vi "Catapult Controller.vi"(8 "error in (no error)":errorcluster, 9 "De-energize w/out Re-energizing":bool, 10 "Wedge Button":bool, 11 "Catapult Trigger":bool) -> (0 "error out":errorcluster)   [LabVIEW 2013]
uses:
  Systems/Catapult/Catapult.lvclass
  Robot Global Data.vi
  Commands/CT-Energize-Cmd/CT-Energize-Cmd.lvclass
  <vilib>/Rock Robotics/WPI/Solenoid/WPI_SolenoidSetEnum.vi
  <vilib>/Rock Robotics/WPI/Solenoid/WPI_SolenoidValue.ctl
  Commands/CT-Stop-Command/CT-Stop-Cmd.lvclass
  Commands/CT-De-energize-Command/CT-De-energize-Cmd.lvclass
panel:
  in  "Boolean 4":bool
  in  "Boolean 3":bool
  in  "Counter":i8
  # "Disabled (Used in Testing)"
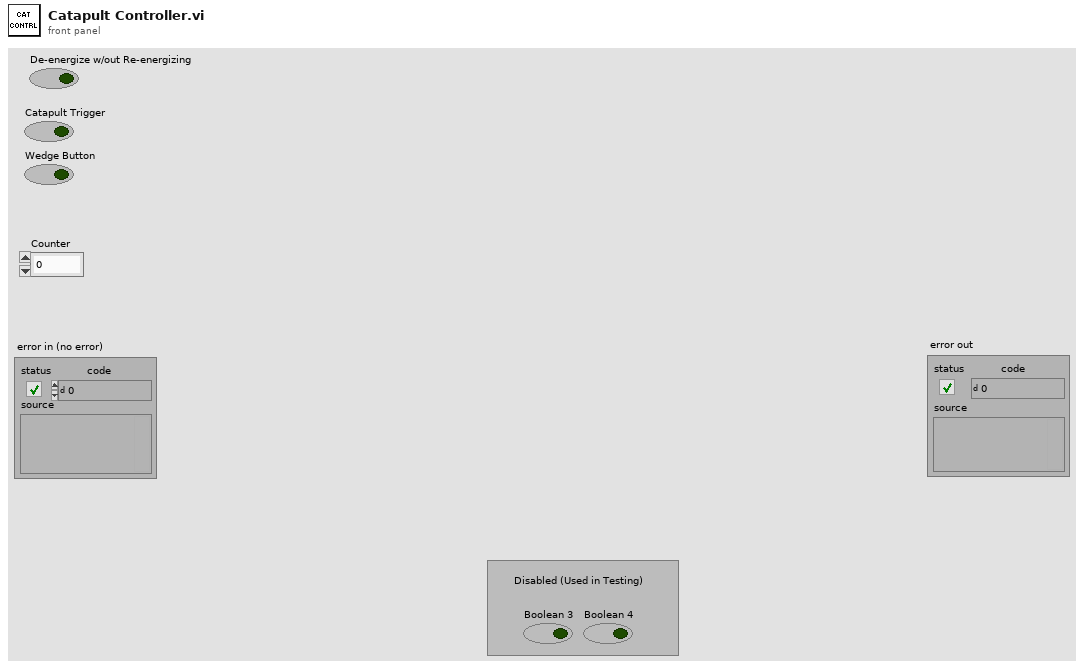
[diagram p1: front panel]
types:
  T1 = typedef "Semaphore RefNum" = refnum<k1>
  T2 = typedef "WPI_DigitalInputDevRef.ctl" = cluster{"DevStatus":errorcluster, "DIO Channel":T3, "Digital Module":T4}
  T3 = typedef "FPGA_DIOChannel.ctl" = enum8{"DIO 1", "DIO 2", "DIO 3", "DIO 4", "DIO 5", "DIO 6", "DIO 7", "DIO 8", "DIO 9", "DIO 10", "DIO 11", "DIO 12", "DIO 13", "DIO 14", "Invalid"}
  T4 = typedef "FPGA_TypedefDigitalModule.ctl" = enum16{"Digital Module 1", "Digital Module 2"}
  T5 = typedef "WPI_SolenoidValue.ctl" = enum16{"Off", "On", "Forward", "Reverse"}
  T6 = typedef "WPI_SolenoidDevRef.ctl" = cluster{"DevStatus":errorcluster, "Solenoid Module":T7, "Forward Solenoid Channel":T8, "Reverse Solenoid Channel":T8}
  T7 = typedef "FPGA_TypedefSolenoidModule.ctl" = enum16{"Solenoid Module 1", "Solenoid Module 2"}
  T8 = typedef "WPI_SolenoidChannel.ctl" = enum8{"Solenoid 1", "Solenoid 2", "Solenoid 3", "Solenoid 4", "Solenoid 5", "Solenoid 6", "Solenoid 7", "Solenoid 8", "Invalid"}
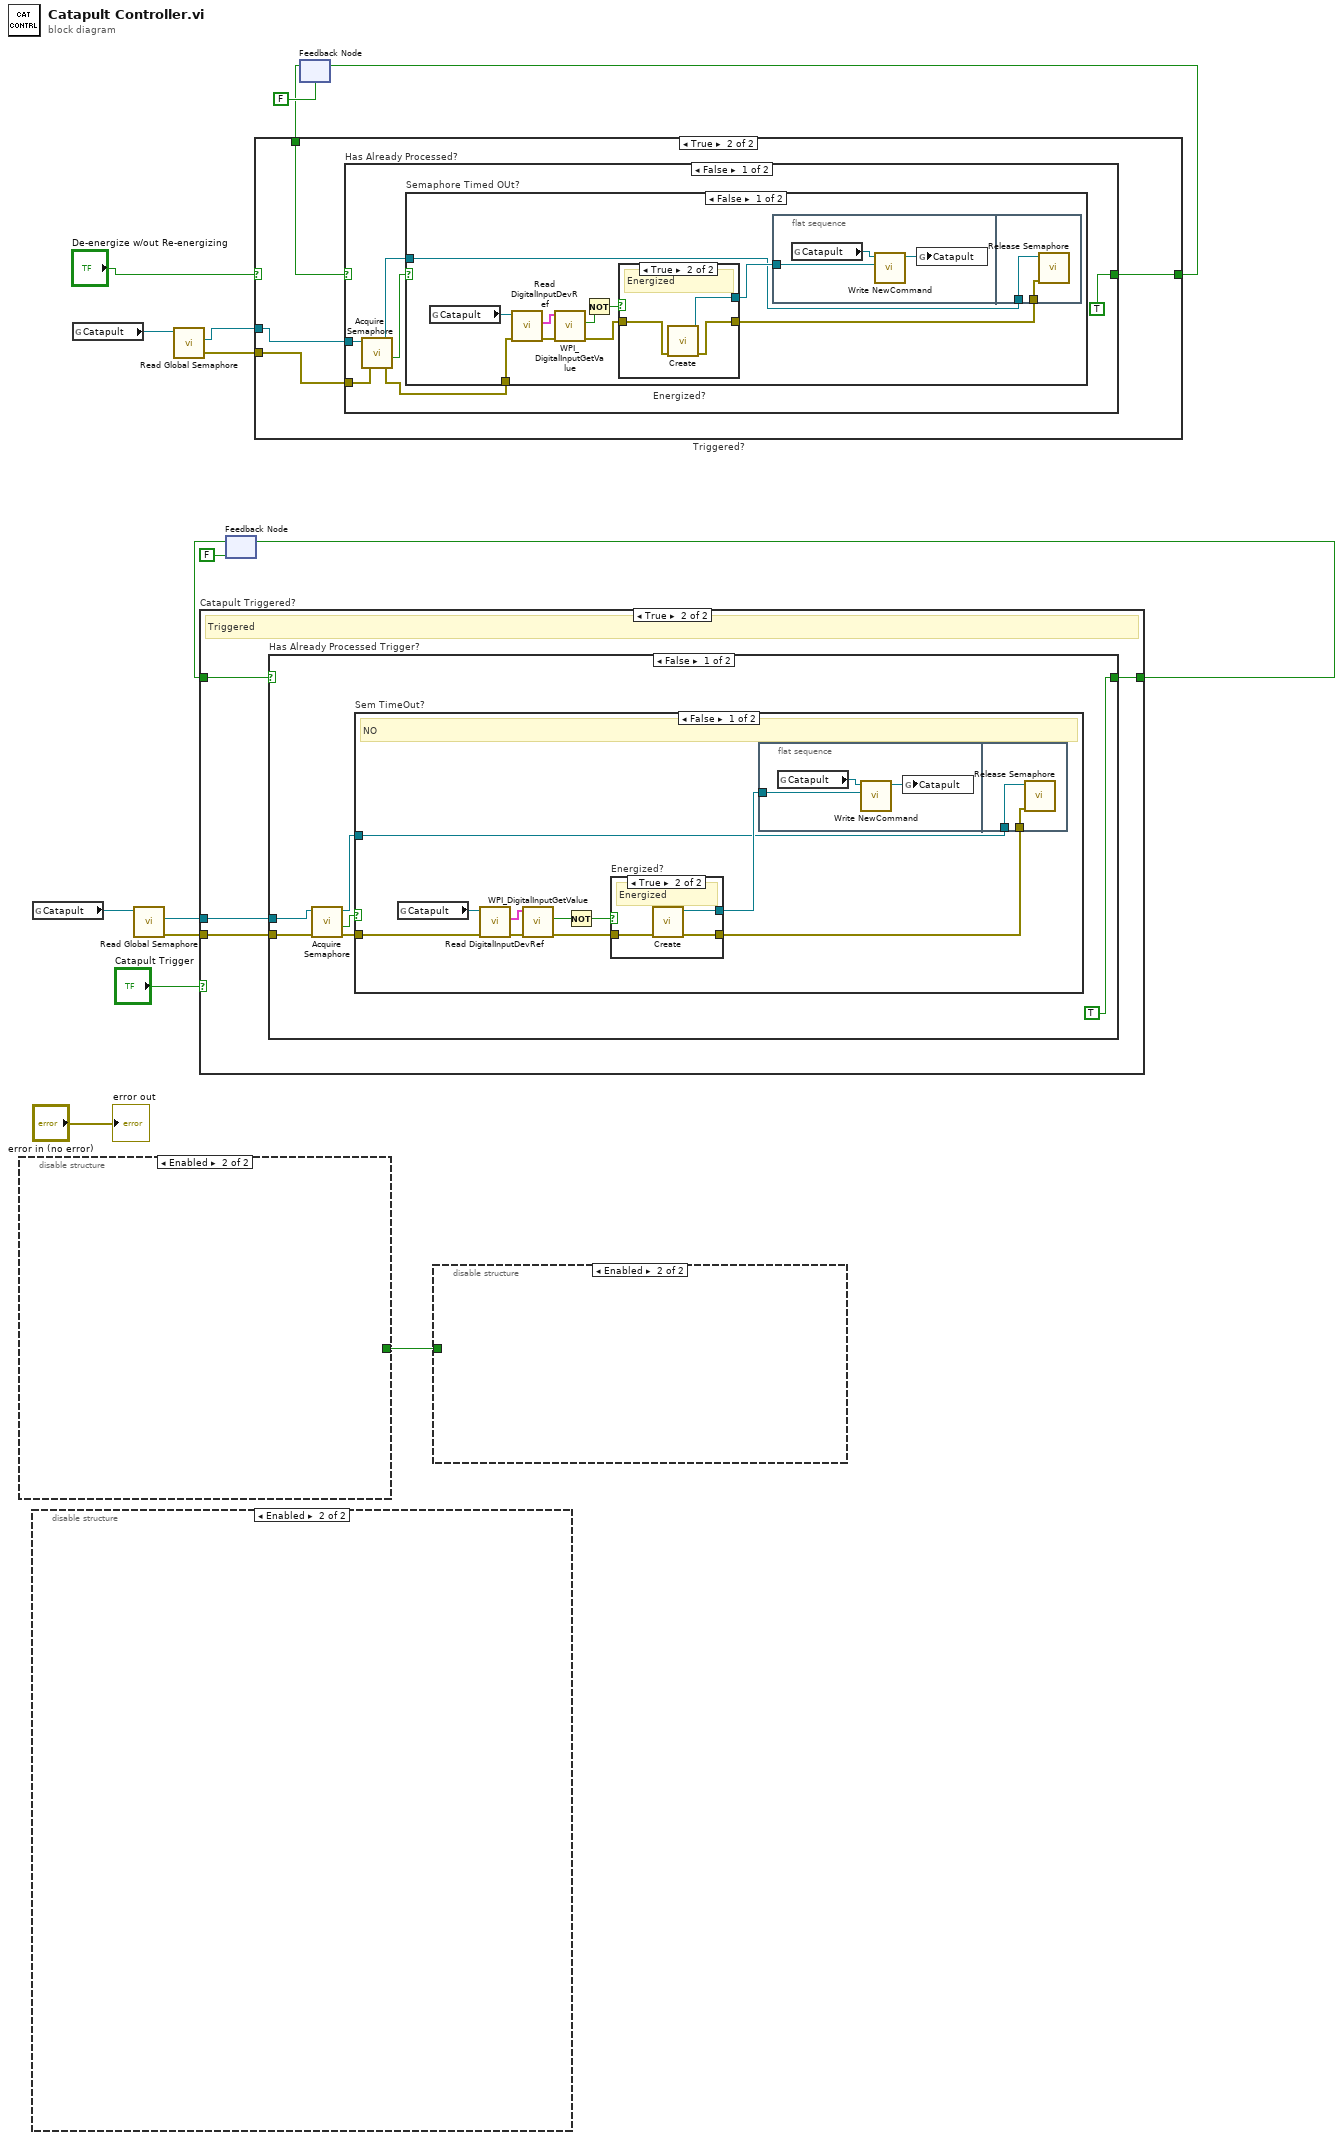
[diagram p0: block diagram]
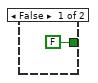
[diagram p2: hidden frame]
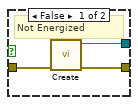
[diagram p3: hidden frame]
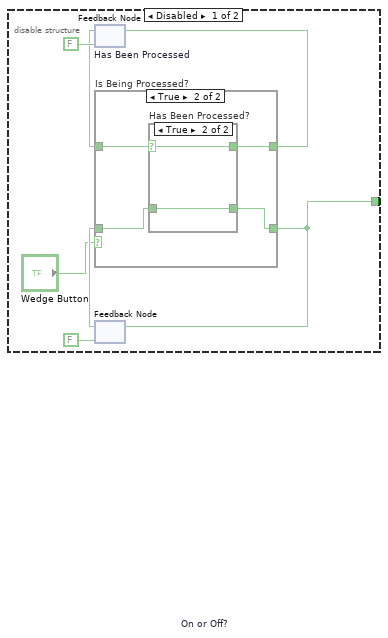
[diagram p6: hidden frame]
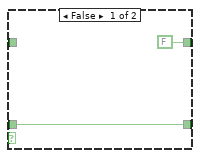
[diagram p7: hidden frame]
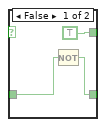
[diagram p8: hidden frame]
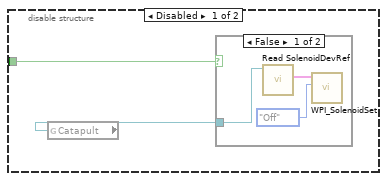
[diagram p9: hidden frame]
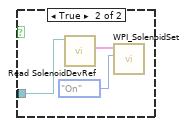
[diagram p10: hidden frame]
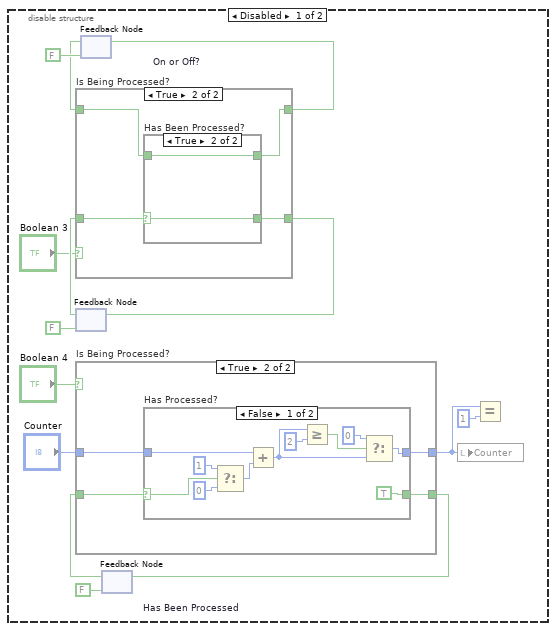
[diagram p11: hidden frame]
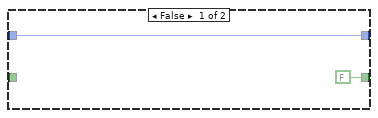
[diagram p12: hidden frame]
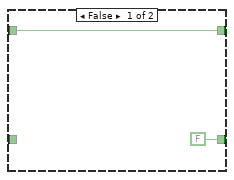
[diagram p14: hidden frame]
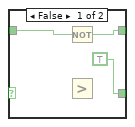
[diagram p15: hidden frame]
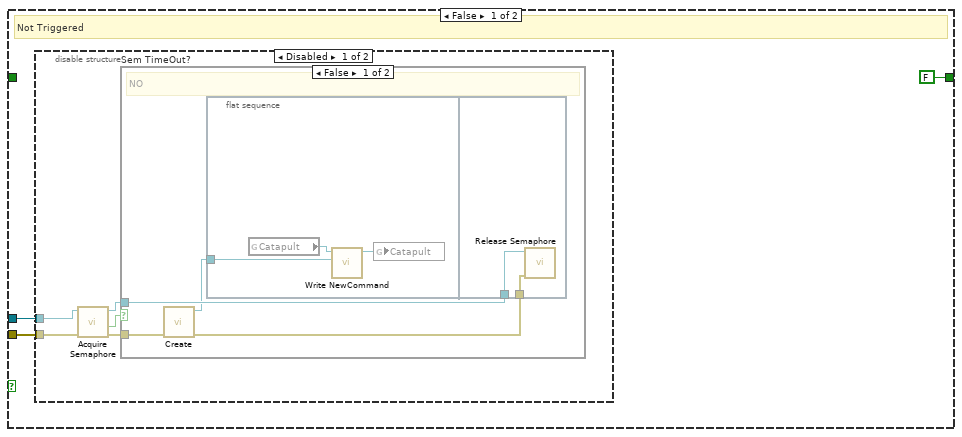
[diagram p16: hidden frame]
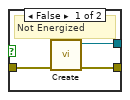
[diagram p19: hidden frame]
diagram:
  n1 = disable-structure shown="Enabled" {
    disable-tunnel: [w17 _] -> w8
    frame Disabled {
      n2 = feedback #1 "Has Been Processed"(FALSE) -> (w22:bool)
      n3 = feedback #2 "On or Off?"(FALSE) -> (w19:bool)
      n4 = case "Is Being Processed?" shown="True" "Wedge Button" {
        tunnel: w22 -> [_ w29]
        tunnel: [FALSE w28] -> w21
        tunnel: w19 -> [w24 w27]
        tunnel: [w24 w26] -> w17
        frame False {
        }
        frame True {
          n5 = case "Has Been Processed?" shown="True" w29 {
            selector: w29 -> [_ w34]
            tunnel: [TRUE w34] -> w28
            tunnel: w27 -> [w31 w33]
            tunnel: [w30 w33] -> w26
            frame False {
              n6 = Not(x=w31) -> (.not. x?=w30:bool)
            }
            frame True {
            }
          }
        }
      }
      n7 = feedback-in #1(w21) -> ()
      n8 = feedback-in #2(w17) -> ()
    }
    frame Enabled {
    }
  }
  n9 = global read "Robot Global Data.vi" "Catapult"() -> (w15:refnum<class "Catapult.lvclass">)
  n10 = disable-structure shown="Enabled" {
    frame Disabled {
      n11 = feedback #3 "Has Been Processed"(FALSE) -> (w47:bool)
      n12 = feedback #4 "On or Off?"(FALSE) -> (w43:bool)
      n13 = case "Is Being Processed?" shown="True" "Boolean 3" {
        tunnel: w47 -> [_ w73]
        tunnel: [FALSE w72] -> w46
        tunnel: w43 -> [w68 w71]
        tunnel: [w68 w70] -> w42
        frame False {
        }
        frame True {
          n14 = case "Has Been Processed?" shown="True" w73 {
            selector: w73 -> [_ w78]
            tunnel: [TRUE w78] -> w72
            tunnel: w71 -> [w75 w77]
            tunnel: [w74 w77] -> w70
            frame False {
              n15 = Not(x=w75) -> (.not. x?=w74:bool)
              n16 = Greater?() -> ()  [unwired: 2 in, 1 out]
            }
            frame True {
            }
          }
        }
      }
      n17 = feedback-in #3(w46) -> ()
      n18 = feedback-in #4(w42) -> ()
      n19 = feedback #5(FALSE) -> (w39:bool)
      n20 = case "Is Being Processed?" shown="True" "Boolean 4" {
        tunnel: "Counter" -> [w49 w54]
        tunnel: [w49 w53] -> w37
        tunnel: w39 -> [_ w52]
        tunnel: [FALSE w51] -> w38
        frame False {
        }
        frame True {
          n21 = case "Has Processed?" shown="False" w52 {
            selector: w52 -> [w64 w66]
            tunnel: w54 -> [w65 w67]
            tunnel: [w56 w67] -> w53
            tunnel: [TRUE w66] -> w51
            frame False {
              n22 = Select(t=i8 1, s=w64, f=i8 0) -> (s? t:f=w61:i8)
              n23 = Add(x=w65, y=w61) -> (x+y=w57:i8)
              n24 = Greater Or Equal?(x=w57, y=i8 2) -> (x >= y?=w59:bool)
              n25 = Select(t=i8 0, s=w59, f=w57) -> (s? t:f=w56:i8)
            }
            frame True {
            }
          }
        }
      }
      n26 = feedback-in #5(w38) -> ()
      n27 = local write "Counter"(w37) -> ()
      n28 = Equal?(x=w37, y=i8 1) -> ()  [unwired: 1 out]
    }
    frame Enabled {
    }
  }
  n29 = global read "Robot Global Data.vi" "Catapult"() -> (w4:refnum<class "Catapult.lvclass">)
  n30 = call-dynamic "Read Global Semaphore.vi"("System in"=w15) -> ("error out"=w13:errorcluster, "semaphore"=w14:T1)  [unwired: 8 in, 1 out]
  n31 = call-dynamic "Read Global Semaphore.vi"("System in"=w4) -> ("error out"=w1:errorcluster, "semaphore"=w2:T1)  [unwired: 8 in, 1 out]
  n32 = feedback #6(FALSE) -> (w10:bool)
  n33 = case "Catapult Triggered?" shown="True" "Catapult Trigger" {
    tunnel: w14 -> [w81 w99]
    tunnel: w13 -> [w80 w98]
    tunnel: w10 -> [_ w97]
    tunnel: [FALSE w96] -> w9
    frame False {
      # "Not Triggered"
      n34 = disable-structure shown="Disabled" {
        disable-tunnel: w81 -> [w83 _]
        disable-tunnel: w80 -> [w82 _]
        frame Disabled {
          n35 = call <vilib>:"Acquire Semaphore.vi"("error in (no error)"=w82, "semaphore"=w83) -> ("error out"=w85:errorcluster, "timed out"=w84:bool, "semaphore out"=w86:T1)  [unwired: 3 in]
          n36 = case "Sem TimeOut?" shown="False" w84 {
            tunnel: w85 -> [w89 _]
            tunnel: w86 -> [w90 _]
            frame False {
              # "NO"
              n37 = call "Create.vi"("error in (no error)"=w89) -> ("error out"=w88:errorcluster, "CT-Stop-Cmd.lvclass"=w87:refnum<class "CT-Stop-Cmd.lvclass">)  [unwired: 8 in]
              n38 = flat-sequence {
                tunnel: w87 -> [w91]
                tunnel: w88 -> [w95]
                tunnel: w90 -> [w94]
                frame #0 {
                  n39 = global read "Robot Global Data.vi" "Catapult"() -> (w93:refnum<class "Catapult.lvclass">)
                  n40 = call-dynamic "Write NewCommand.vi"("Command.lvclass"=w91, "System in"=w93) -> ("System out"=w92:refnum<class "Catapult.lvclass">)  [unwired: 8 in, 1 out]
                  n41 = global write "Robot Global Data.vi" "Catapult"(w92) -> ()
                }
                frame #1 {
                  n42 = call <vilib>:"Release Semaphore.vi"("error in (no error)"=w95, "semaphore"=w94) -> ()  [unwired: 4 in, 2 out]
                }
              }
            }
            frame True {
              # "YES"
            }
          }
        }
        frame Enabled {
        }
      }
    }
    frame True {
      # "Triggered"
      n43 = case "Has Already Processed Trigger?" shown="False" w97 {
        selector: w97 -> [_ w127]
        tunnel: w99 -> [w105 _]
        tunnel: w98 -> [w101 _]
        tunnel: [TRUE w127] -> w96
        frame False {
          n44 = call <vilib>:"Acquire Semaphore.vi"("error in (no error)"=w101, "semaphore"=w105) -> ("error out"=w103:errorcluster, "timed out"=w104:bool, "semaphore out"=w102:T1)  [unwired: 3 in]
          n45 = case "Sem TimeOut?" shown="False" w104 {
            tunnel: w103 -> [w109 _]
            tunnel: w102 -> [w114 _]
            frame False {
              # "NO"
              n46 = global read "Robot Global Data.vi" "Catapult"() -> (w112:refnum<class "Catapult.lvclass">)
              n47 = call-dynamic "Read DigitalInputDevRef.vi"("error in (no error)"=w109, "Catapult in"=w112) -> ("error out"=w111:errorcluster, "DigitalInputDevRef"=w113:T2)  [unwired: 7 in, 1 out]
              n48 = call <vilib>:"WPI_DigitalInputGetValue.vi"("error in (no error)"=w111, "DigitalInputDevRef"=w113) -> ("error out"=w110:errorcluster, "Value"=w107:bool)  [unwired: 7 in, 1 out]
              n49 = Not(x=w107) -> (.not. x?=w106:bool)
              n50 = case "Energized?" shown="True" w106 {
                tunnel: [w123 w126] -> w115
                tunnel: w110 -> [w122 w124]
                tunnel: [w121 w125] -> w108
                frame False {
                  # "Not Energized"
                  n51 = call "Create.vi"("error in (no error)"=w122) -> ("error out"=w121:errorcluster, "CT-Energize-Cmd.lvclass"=w123:refnum<class "CT-Energize-Cmd.lvclass">)  [unwired: 9 in]
                }
                frame True {
                  # "Energized"
                  n52 = call "Create.vi"("error in (no error)"=w124) -> ("error out"=w125:errorcluster, "CT-De-energize-Cmd.lvclass"=w126:refnum<class "CT-De-energize-Cmd.lvclass">)  [unwired: 9 in]
                }
              }
              n53 = flat-sequence {
                tunnel: w115 -> [w116]
                tunnel: w108 -> [w120]
                tunnel: w114 -> [w119]
                frame #0 {
                  n54 = global read "Robot Global Data.vi" "Catapult"() -> (w118:refnum<class "Catapult.lvclass">)
                  n55 = call-dynamic "Write NewCommand.vi"("Command.lvclass"=w116, "System in"=w118) -> ("System out"=w117:refnum<class "Catapult.lvclass">)  [unwired: 8 in, 1 out]
                  n56 = global write "Robot Global Data.vi" "Catapult"(w117) -> ()
                }
                frame #1 {
                  n57 = call <vilib>:"Release Semaphore.vi"("error in (no error)"=w120, "semaphore"=w119) -> ()  [unwired: 4 in, 2 out]
                }
              }
            }
            frame True {
              # "YES"
            }
          }
        }
        frame True {
        }
      }
    }
  }
  n58 = feedback-in #6(w9) -> ()
  n59 = feedback #7(FALSE) -> (w6:bool)
  n60 = case "Triggered?" shown="True" "De-energize w/out Re-energizing" {
    tunnel: w6 -> [_ w132]
    tunnel: [FALSE w131] -> w5
    tunnel: w2 -> [_ w129]
    tunnel: w1 -> [_ w130]
    frame False {
    }
    frame True {
      n61 = case "Has Already Processed?" shown="False" w132 {
        selector: w132 -> [_ w160]
        tunnel: [TRUE w160] -> w131
        tunnel: w130 -> [w137 _]
        tunnel: w129 -> [w136 _]
        frame False {
          n62 = call <vilib>:"Acquire Semaphore.vi"("error in (no error)"=w137, "semaphore"=w136) -> ("error out"=w134:errorcluster, "timed out"=w135:bool, "semaphore out"=w133:T1)  [unwired: 3 in]
          n63 = case "Semaphore Timed OUt?" shown="False" w135 {
            tunnel: w134 -> [w142 _]
            tunnel: w133 -> [w139 _]
            frame False {
              n64 = global read "Robot Global Data.vi" "Catapult"() -> (w148:refnum<class "Catapult.lvclass">)
              n65 = call-dynamic "Read DigitalInputDevRef.vi"("error in (no error)"=w142, "Catapult in"=w148) -> ("error out"=w143:errorcluster, "DigitalInputDevRef"=w147:T2)  [unwired: 7 in, 1 out]
              n66 = call <vilib>:"WPI_DigitalInputGetValue.vi"("error in (no error)"=w143, "DigitalInputDevRef"=w147) -> ("error out"=w146:errorcluster, "Value"=w144:bool)  [unwired: 7 in, 1 out]
              n67 = Not(x=w144) -> (.not. x?=w145:bool)
              n68 = case "Energized?" shown="True" w145 {
                tunnel: [w156 w157] -> w141
                tunnel: w146 -> [w155 w159]
                tunnel: [w154 w158] -> w140
                frame False {
                  # "Not Energized"
                  n69 = call "Create.vi"("error in (no error)"=w155) -> ("error out"=w154:errorcluster, "CT-Energize-Cmd.lvclass"=w156:refnum<class "CT-Energize-Cmd.lvclass">)  [unwired: 9 in]
                }
                frame True {
                  # "Energized"
                  n70 = call "Create.vi"("error in (no error)"=w159) -> ("error out"=w158:errorcluster, "CT-De-energize-Cmd.lvclass"=w157:refnum<class "CT-De-energize-Cmd.lvclass">)  [unwired: 9 in]
                }
              }
              n71 = flat-sequence {
                tunnel: w141 -> [w149]
                tunnel: w140 -> [w153]
                tunnel: w139 -> [w152]
                frame #0 {
                  n72 = global read "Robot Global Data.vi" "Catapult"() -> (w151:refnum<class "Catapult.lvclass">)
                  n73 = call-dynamic "Write NewCommand.vi"("Command.lvclass"=w149, "System in"=w151) -> ("System out"=w150:refnum<class "Catapult.lvclass">)  [unwired: 8 in, 1 out]
                  n74 = global write "Robot Global Data.vi" "Catapult"(w150) -> ()
                }
                frame #1 {
                  n75 = call <vilib>:"Release Semaphore.vi"("error in (no error)"=w153, "semaphore"=w152) -> ()  [unwired: 4 in, 2 out]
                }
              }
            }
            frame True {
            }
          }
        }
        frame True {
        }
      }
    }
  }
  n76 = feedback-in #7(w5) -> ()
  n77 = disable-structure shown="Enabled" {
    disable-tunnel: w8 -> [w161 _]
    frame Disabled {
      n78 = global read "Robot Global Data.vi" "Catapult"() -> (w162:refnum<class "Catapult.lvclass">)
      n79 = case shown="False" w161 {
        tunnel: w162 -> [w165 w168]
        frame False {
          n80 = call-dynamic "Read SolenoidDevRef.vi"("Catapult in"=w165) -> ("SolenoidDevRef"=w164:T6)  [unwired: 8 in, 2 out]
          n81 = call-poly <vilib>:"WPI_SolenoidSet.vi"("Value"=WPI_SolenoidValue."Off", "SolenoidDevRef"=w164) -> ()  [unwired: 8 in, 2 out]
        }
        frame True {
          n82 = call-dynamic "Read SolenoidDevRef.vi"("Catapult in"=w168) -> ("SolenoidDevRef"=w167:T6)  [unwired: 8 in, 2 out]
          n83 = call-poly <vilib>:"WPI_SolenoidSet.vi"("Value"=WPI_SolenoidValue."On", "SolenoidDevRef"=w167) -> ()  [unwired: 8 in, 2 out]
        }
      }
    }
    frame Enabled {
    }
  }
  "error out" <- "error in (no error)"
